vi "Create Default Attributes.vi"(5 "Unique ID":string, 11 "iProcess Step Model in":refnum<class "iProcess Step Model.lvclass">) -> (3 "iProcess Step Model out":refnum<class "iProcess Step Model.lvclass">)   [LabVIEW 2017, in "iProcess Step Model.lvlib" / "iProcess Step Model.lvclass"]
uses:
  iProcess Step Model.lvclass
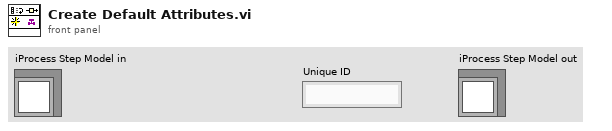
[diagram p1: front panel]
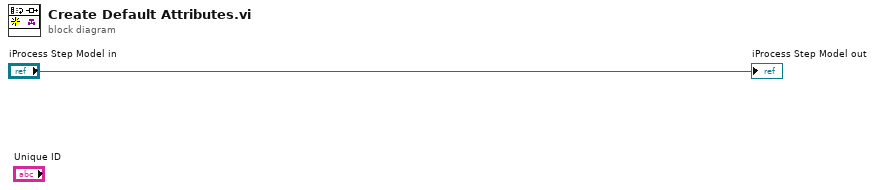
[diagram p0: block diagram]
diagram:
  "iProcess Step Model out" <- "iProcess Step Model in"
